vi "gui-is-detector-possible.vi"(1 "disabled detectors":i32[](array[numeric]), 2 "detector-in":u16(ring) caption="Camera" items=["Newton", "iDus", "Clara", "Xeva"], 3 "enabled detectors":i32[](array[numeric])) -> (0 "detector-out":u16(ring) caption="Camera" items=["Newton", "iDus", "Clara", "Xeva"])   [LabVIEW 2015]
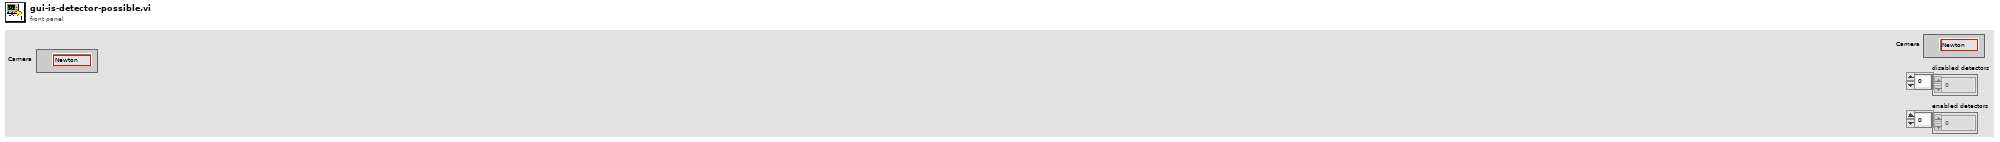
[diagram p1: front panel]
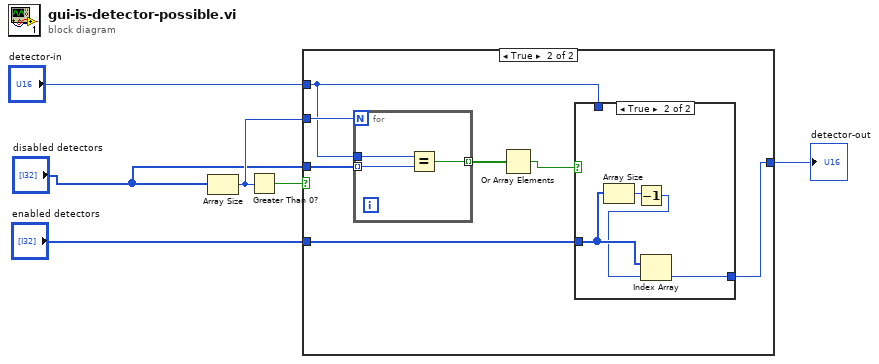
[diagram p0: block diagram]
diagram:
  n1 = Array Size(array="disabled detectors") -> (size(s)=w5:i32)
  n2 = Greater Than 0?(x=w5) -> (x > 0?=w6:bool)
  n3 = case shown="True" w6 {
    tunnel: w5 -> [_ w14]
    tunnel: "disabled detectors" -> [_ w13]
    tunnel: "detector-in" -> [w7 w8]
    tunnel: [w7 w9] -> w2
    tunnel: "enabled detectors" -> [_ w10]
    frame False {
    }
    frame True {
      n4 = for {
        N: w14 -> [_]
        tunnel: w13 -> [w22] mode=indexing
        tunnel: w8 -> [w21]
        tunnel: [w20] -> w12 mode=indexing
        n5 = Equal?(x=w21, y=w22) -> (x = y?=w20:bool)
      }
      n6 = Or Array Elements(Boolean array=w12) -> (logical OR=w11:bool)
      n7 = case shown="True" w11 {
        tunnel: w10 -> [_ w18]
        tunnel: [w15 w19] -> w9
        tunnel: w8 -> [w15 _]
        frame False {
        }
        frame True {
          n8 = Array Size(array=w18) -> (size(s)=w17:i32)
          n9 = Decrement(x=w17) -> (x-1=w16:i32)
          n10 = Index Array "Index Array"(array=w18, index=w16) -> (element=w19:i32)
        }
      }
    }
  }
  "detector-out" <- w2
